vi "TB-Save SPL History.vi"(0 "state":T5, 1 "Log in":T3, 5 "XYGraph in":refnum<vi>, 7 "date/time string":string, 9 "history":cluster{dbl[], dbl[]}[](array[cluster]), 12 "Exposure parameters":T1={"Low cutoff (kHz)"=8.0, "High cutoff (kHz)"=16.0, "Duration (min)"=120.0, "dB SPL"=100.0, "Waveform"=enum."Noise", "WAVfile"=path "", "refWav"=path "", "use mic correction"=FALSE, "micCorrFile"=path "", "Pistonphone Level (dB SPL)"=0.0, "Sampling rate (Hz)"=0.0, "Buffer length (s)"=0.0, "Stream mic"=FALSE, "Fine adjust"={"Max"=0.0, "Min"=0.0}, "Mic gain"=0.0, "atten"=0.0, "resol (Hz)"=0.0, "navgs"=0, "Allow Slack"=FALSE, "max starts"=0, "Freq (kHz)"=8.0, "Tma (s)"=0.0, "Streamed"=[], "Drive"=""}) -> (15 "error out":errorcluster)   [LabVIEW 2020]
uses:
  Typedefs/TB-Runtime state.ctl
  <vilib>/sound2/lvsound2.llb/Sound File Refnum.ctl
  Typedefs/TB-Setup Log.ctl
  Typedefs/TB-Log.ctl
  Typedefs/TB-Slack State.ctl
  Typedefs/TB-Parameters.ctl
  epl-vi-lib/Signal Synthesis VIs/Controls/Waveform XCtl/Waveform Enum.ctl
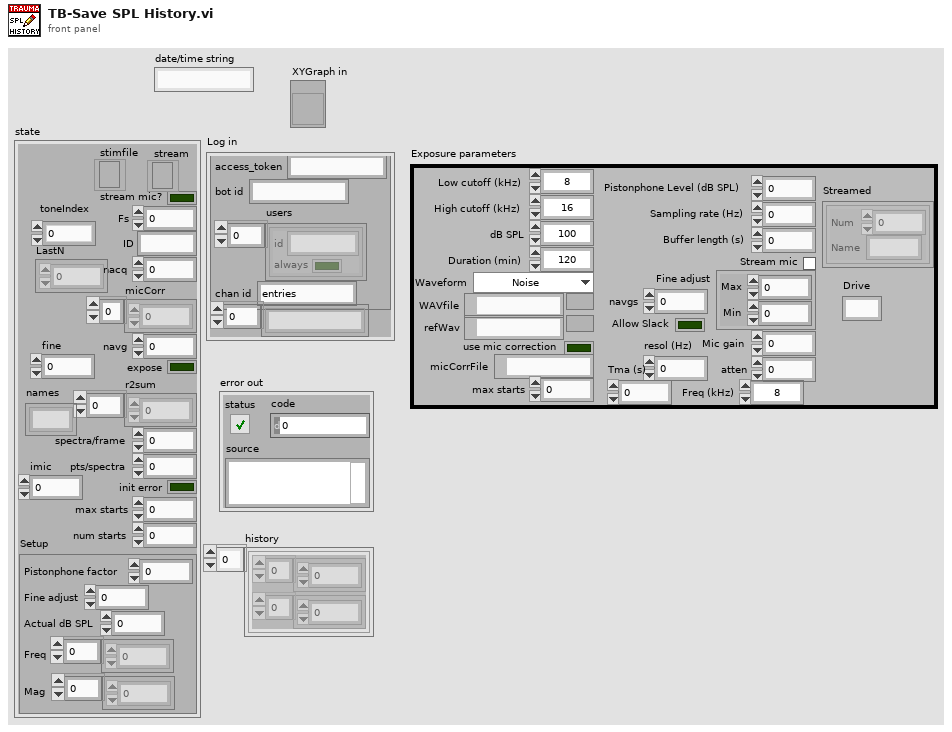
[diagram p1: front panel]
types:
  T1 = typedef "TB-Parameters.ctl" = cluster{"Low cutoff (kHz)":dbl, "High cutoff (kHz)":dbl, "Duration (min)":dbl, "dB SPL":dbl, "Waveform":T2, "WAVfile":path, "refWav":path, "use mic correction":bool, "micCorrFile":path, "Pistonphone Level (dB SPL)":dbl, "Sampling rate (Hz)":dbl, "Buffer length (s)":dbl, "Stream mic":bool, "Fine adjust":cluster{"Max":dbl, "Min":dbl}, "Mic gain":dbl, "atten":dbl, "resol (Hz)":dbl, "navgs":i32, "Allow Slack":bool, "max starts":i32, "Freq (kHz)":dbl, "Tma (s)":dbl, "Streamed":cluster{"Num":i32, "Name":string}[], "Drive":string}
  T2 = typedef "Waveform Enum.ctl" = enum16{"OFF", "Tone", "Noise", "Pulse Train", "File", "FM Sweep", "Chirp Train", "Complex Tone", "FM Tone", "Moving Ripple"}
  T3 = typedef "TB-Log.ctl" = cluster{"Slack":T4, "entries":string[]}
  T4 = typedef "TB-Slack State.ctl" = cluster{"access_token":string, "bot id":string, "users":cluster{"id":string, "always":bool}[], "chan id":string}
  T5 = typedef "TB-Runtime state.ctl" = cluster{"stimfile":T6, "stream mic?":bool, "Fs":dbl, "ID":string, "micCorr":dbl[], "navg":i32, "r2sum":dbl[], "expose":bool, "spectra/frame":i32, "pts/spectra":i32, "nacq":i32, "init error":bool, "max starts":i32, "num starts":i32, "Setup":T7, "toneIndex":i32, "LastN":dbl[], "fine":dbl, "imic":i32, "stream":refnum<file>, "names":string[]}
  T6 = typedef "Sound File Refnum.ctl" = refnum<file>
  T7 = typedef "TB-Setup Log.ctl" = cluster{"Pistonphone factor":dbl, "Fine adjust":dbl, "Actual dB SPL":dbl, "Freq":dbl[], "Mag":dbl[]}
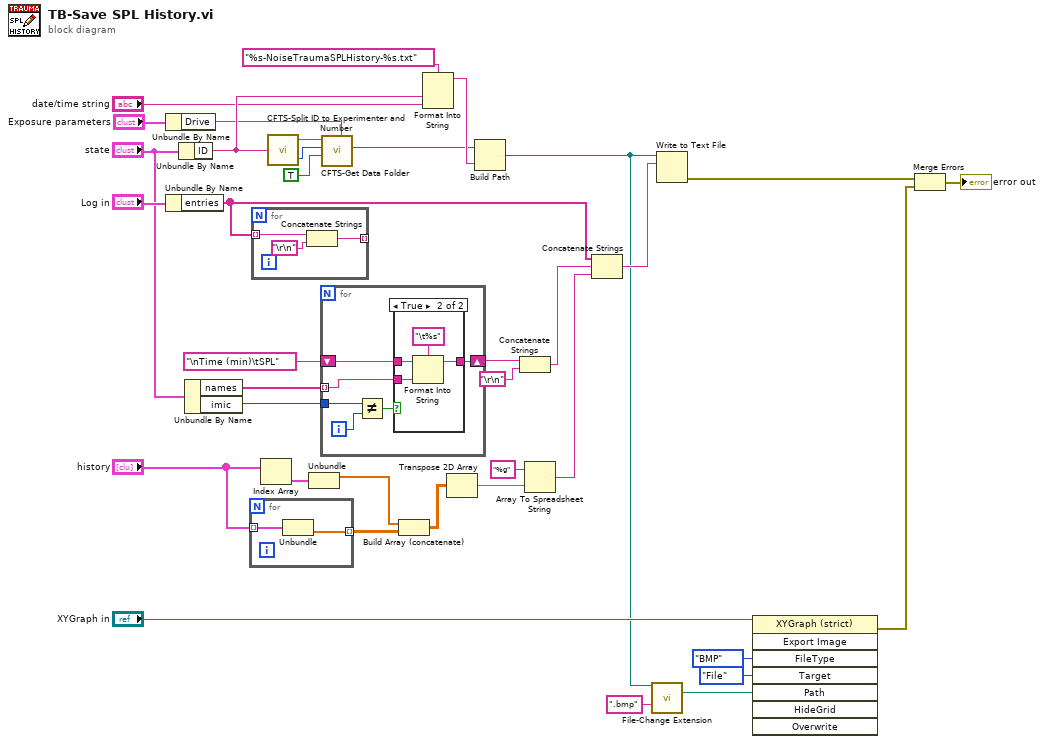
[diagram p0: block diagram]
diagram:
  n1 = Unbundle By Name("Exposure parameters") -> ("Drive"=w1:string)
  n2 = Unbundle By Name("Log in") -> ("entries"=w22:string[])
  n3 = Unbundle By Name("state") -> ("ID"=w33:string)
  n4 = Unbundle By Name("state") -> ("names"=w4:string[], "imic"=w3:i32)
  n5 = for {
    tunnel: "history" -> [w39] mode=indexing
    tunnel: [w38] -> w32 mode=indexing
    n6 = Unbundle(w39) -> (w38:dbl[])  [unwired: 1 out]
  }
  n7 = for {
    tunnel: w22 -> [w42] mode=indexing
    tunnel: [w40] -> _ mode=indexing
    n8 = Concatenate Strings(w42, "\r\n") -> (w40:string)
  }
  n9 = Index Array(array="history") -> (element=w11:cluster{dbl[], dbl[]})  [unwired: 1 in]
  n10 = call "CFTS-Split ID to Experimenter and Number.vi"("ID"=w33) -> ("Experimenter"=w36:string, "Number"=w37:i32)
  n11 = Unbundle(w11) -> (w10:dbl[])  [unwired: 1 out]
  n12 = for {
    shift-right: [w47] -> w7
    shift-left: "\nTime (min)\tSPL" ("string") -> [w48]
    tunnel: w4 -> [w46] mode=indexing
    tunnel: w3 -> [w45]
    i -> [w44]
    n13 = Not Equal?(x=w45, y=w44) -> (x != y?=w43:bool)
    n14 = case shown="True" w43 {
      tunnel: w48 -> [w49 w53]
      tunnel: [w49 w52] -> w47
      tunnel: w46 -> [_ w51]
      frame False {
      }
      frame True {
        n15 = Format Into String(format string="\t%s", initial string=w53, w51) -> (resulting string=w52:string)  [unwired: 1 in, 1 out]
      }
    }
  }
  n16 = call "CFTS-Get Data Folder.vi"("Drive"=w1, "create?"=TRUE, "Number"=w37, "Experimenter"=w36) -> ("Data folder"=w25:path)  [unwired: 6 in, 1 out]
  n17 = Build Array (concatenate)(w10, w32) -> (w31:dbl[][])
  n18 = Format Into String(format string="%s-NoiseTraumaSPLHistory-%s.txt", w33, "date/time string") -> (resulting string=w34:string)  [unwired: 2 in, 1 out]
  n19 = Transpose 2D Array(2D array=w31) -> (transposed array=w30:dbl[][])
  n20 = Build Path(base path=w25, name or relative path=w34) -> (appended path=w18:path)
  n21 = Concatenate Strings(w7, "\r\n") -> (w6:string)
  n22 = Array To Spreadsheet String(array=w30, 3:"%g" ("format string")) -> (spreadsheet string=w28:string)  [unwired: 1 in]
  n23 = Concatenate Strings(w22, w6, w28) -> (w27:string)
  n24 = call "File-Change Extension.vi"("Path"=w18, "new extension"=".bmp") -> ("new path"=w17:path)  [unwired: 13 in]
  n25 = Write to Text File(file (use dialog)=w18, text=w27) -> (error out=w26:errorcluster)  [unwired: 2 in, 2 out]
  n26 = invoke class="XYGraph (strict)" method="Export Image"(reference="XYGraph in", "FileType"=enum32{"BMP", "EPS", "EMF", "PICT"}."BMP" ("File Type"), "Target"=enum32{"File", "Clipboard"}."File", "Path"=w17) -> (error out=w13:errorcluster)  [unwired: 4 in, 7 out]
  n27 = Merge Errors(w26, w13) -> (→"error out":errorcluster)
